vi "mod_Rician Selective Fading (Gans).vi"(0 "profile length (samples)":i32=1000, 1 "rician parameter K (dB)":dbl=2.0 format="%.2f", 2 "number of paths":i32, 5 "sampling frequency (Hz)":dbl=1.0 format="%.2f", 7 "doppler spread (Hz)":dbl=0.01 format="%.2p", 9 "seed in (0xFFFFFFFF)":i32=-1 format="%.0x", 11 "error in (no error)":errorcluster, 12 "fading variance":dbl=1.0 format="%.2f", 13 "reset? (T)":bool=TRUE) -> (4 "Rician Fading profile":cdb[][](array[numeric]), 10 "next seed":i32 format="%.0x", 15 "error out":errorcluster)   [LabVIEW 2020, in "niDMT.lvlib"]
doc: "The Rayleigh fading channel is generated based on Clarke and Gans Model using the Doppler filter with U-shaped power spectral density. \n \n\n Inputs:\n 1) Doppler spread (Hz) \n - range : double precision (default:20)\n - an example : a running vehicle with 65mph (104km/h), the carrier frequency of 900MHz\n The speed of the vehicle = 65*1.6*1000/3600 = 28.89m/s\n Doppler frequency = (900MHz)*(28.89m/s)/(300*10^6m/s) = 86.67 Hz\n 2) Fading variance : the variance of the fading channel output\n - range : double precision (default:2)\n 3) Input waveform : Input signal samples\n - some default values were set.\n (dt:0.00025, the number of samples:4000)\n 4) seed in (0xFFFFFFFF)\n 5) Error in\n\n Outputs:\n 1) Rayleigh fading profile : the complex fading channel output\n 2) Error out"
uses:
  <vilib>/addons/Modulation/niDMT.lvlib
  <vilib>/addons/Modulation/niAMT.lvlib
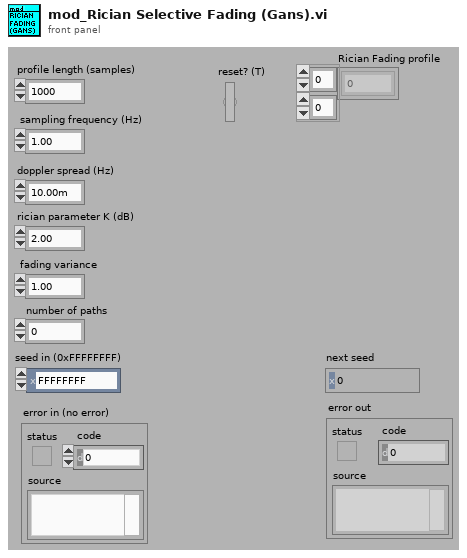
[diagram p1: front panel]
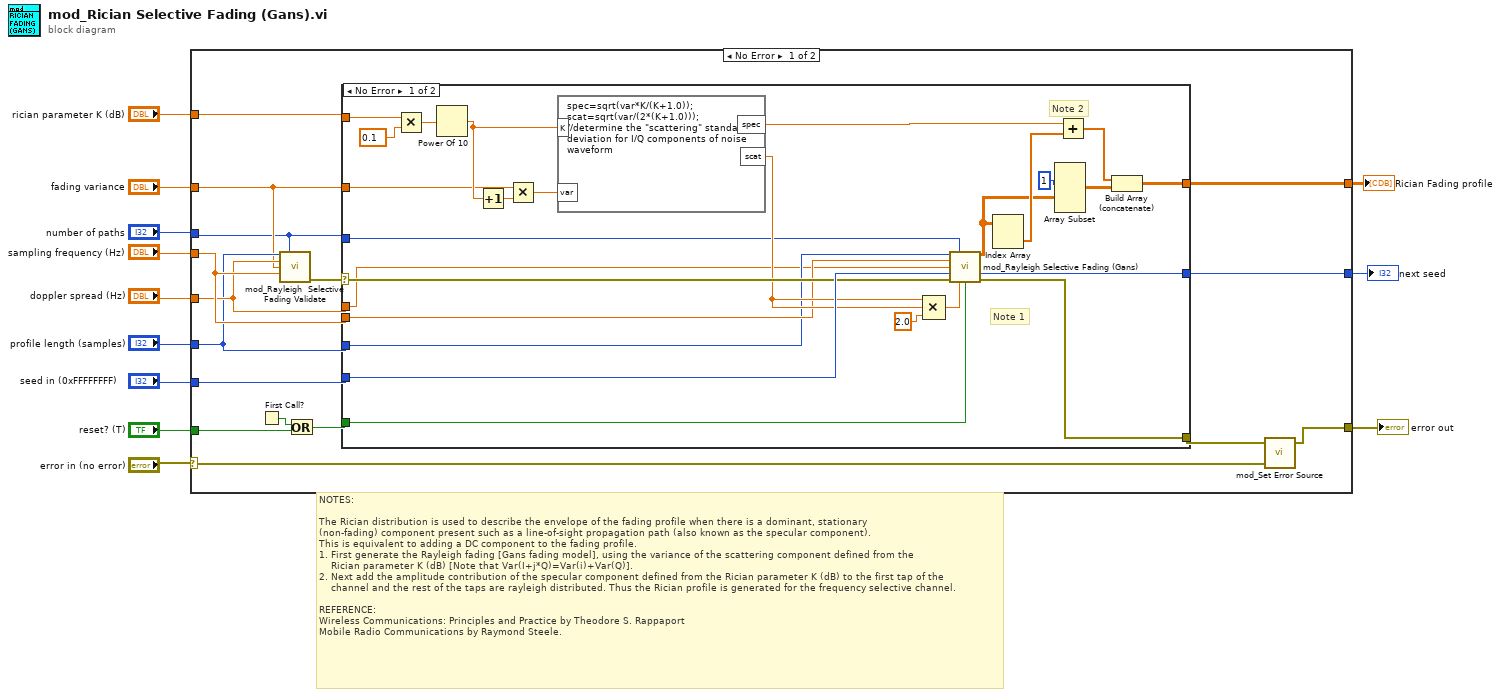
[diagram p0: block diagram]
diagram:
  # "NOTES:\n\nThe Rician distribution is used to describe the envelope of the fading profile when there is a dominant, stationary\n(non-fading) component present such as a line-of-sight propagation path (also known as the specular component).\nThis is equivalent to adding a DC component to the fading profile.\n1. First generate the Rayleigh fading [Gans fading model], using the variance of the scattering component defined from the\n    Rician parameter K (dB) [Note that Var(I+j*Q)=Var(i)+Var(Q)].\n2. Next add the amplitude contribution of the specular component defined from the Rician parameter K (dB) to the first tap of the\n    channel and the rest of the taps are rayleigh distributed. Thus the Rician profile is generated for the frequency selective channel.\n\nREFERENCE:\nWireless Communications: Principles and Practice by Theodore S. Rappaport\nMobile Radio Communications by Raymond Steele."
  n1 = case shown="No Error" "error in (no error)" {
    selector: "error in (no error)" -> [w27 w56]
    tunnel: [w28 w56] -> w12
    tunnel: "rician parameter K (dB)" -> [w15 _]
    tunnel: "fading variance" -> [w16 _]
    tunnel: "sampling frequency (Hz)" -> [w23 _]
    tunnel: "doppler spread (Hz)" -> [w22 _]
    tunnel: "profile length (samples)" -> [w21 _]
    tunnel: "seed in (0xFFFFFFFF)" -> [w20 _]
    tunnel: "reset? (T)" -> [w18 _]
    tunnel: [w17 _] -> w3
    tunnel: "number of paths" -> [w13 _]
    tunnel: [w14 _] -> w1
    frame No Error {
      n2 = First Call?() -> (First Call?: T/F=w19:bool)
      n3 = call <vilib>:"mod_Rayleigh  Selective Fading Validate.vi"("profile length (samples)"=w21, "paths"=w13, "doppler spread (Hz)"=w22, "fading variance"=w16, "sampling frequency"=w23) -> ("error out"=w25:errorcluster)  [unwired: 10 out]
      n4 = Or(x=w19, y=w18) -> (x .or. y?=w24:bool)
      n5 = case shown="No Error" w25 {
        selector: w25 -> [w50 w55]
        tunnel: w22 -> [w30 _]
        tunnel: w21 -> [w38 _]
        tunnel: [w45 w55] -> w26
        tunnel: w20 -> [w51 _]
        tunnel: w23 -> [w39 _]
        tunnel: w15 -> [w52 _]
        tunnel: w24 -> [w46 _]
        tunnel: w16 -> [w42 _]
        tunnel: [w44 _] -> w17
        tunnel: w13 -> [w37 _]
        tunnel: [w31 _] -> w14
        frame No Error {
          # "Note 2"
          # "Note 1"
          n6 = Multiply(x=w52, y=0.1) -> (x*y=w54:dbl)
          n7 = Power Of 10(x=w54) -> (10^x=w43:dbl)
          n8 = Increment(x=w43) -> (x+1=w41:dbl)
          n9 = Multiply(x=w42, y=w41) -> (x*y=w40:dbl)
          n10 = formula code="spec=sqrt(var*K/(K+1.0));\nscat=sqrt(var/(2*(K+1.0)));\n//determine the \"scattering\" standard deviation for I/Q components of noise waveform"("K"=w43, "var"=w40) -> ("scat"=w49:dbl, "spec"=w29:dbl)
          n11 = Compound Arithmetic op=MULTIPLY(w49, w49, 2.0 ("value")) -> (w48:dbl)
          n12 = call <vilib>:"mod_Rayleigh Selective Fading (Gans).vi"("profile length (samples)"=w38, "number of paths"=w37, "sampling frequency (Hz)"=w39, "doppler spread (Hz)"=w30, "seed in (0xFFFFFFFF)"=w51, "error in (no error)"=w50, "fading variance"=w48, "reset? (T)"=w46) -> ("Rayleigh fading profile"=w35:cdb[][], "seed out"=w44:i32, "error out"=w45:errorcluster)  [unwired: 5 out]
          n13 = Index Array(array=w35) -> (element=w36:cdb[])  [unwired: 2 in]
          n14 = Array Subset(array=w35, index (row)=1 ("index")) -> (w32:cdb[][])  [unwired: 3 in]
          n15 = Add(x=w29, y=w36) -> (x+y=w33:cdb[])
          n16 = Build Array (concatenate)(w33, w32) -> (w31:cdb[][])
        }
        frame Error {
        }
      }
      n17 = call <vilib>:"mod_Set Error Source.vi"("initial error in (no error)"=w27, "final error in (no error)"=w26) -> ("error out"=w28:errorcluster)  [unwired: 1 in, 2 out]
    }
    frame Error {
    }
  }
  "error out" <- w12
  "next seed" <- w3
  "Rician Fading profile" <- w1
